vi "quadratic_eq_solve.vi"(2 "C":dbl, 3 "B":dbl, 4 "A":dbl) -> (0 "x2":dbl, 1 "x1":dbl)   [LabVIEW 2018]
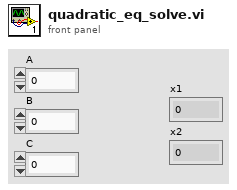
[diagram p1: front panel]
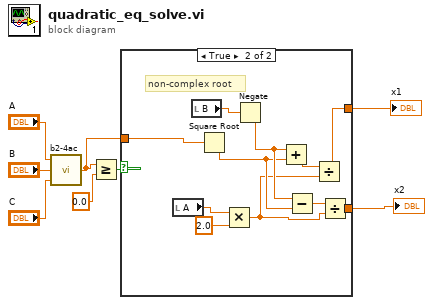
[diagram p0: block diagram]
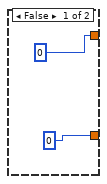
[diagram p2: hidden frame]
diagram:
  n1 = call "b2-4ac.vi"("C"="C", "B"="B", "A"="A") -> ("b2-4ac"=w2:dbl)
  n2 = Greater Or Equal?(x=w2, y=0.0) -> (x >= y?=w5:bool)
  n3 = case shown="True" w5 {
    tunnel: w2 -> [_ w21]
    tunnel: [0 w16] -> w4
    tunnel: [0 w11] -> w3
    frame False {
    }
    frame True {
      # "non-complex root"
      n4 = local read "A"() -> (w19:dbl)
      n5 = local read "B"() -> (w20:dbl)
      n6 = Square Root(x=w21) -> (sqrt(x)=w14:dbl)
      n7 = Multiply(x=w19, y=2.0) -> (x*y=w12:dbl)
      n8 = Negate(x=w20) -> (-x=w15:dbl)
      n9 = Add(x=w15, y=w14) -> (x+y=w17:dbl)
      n10 = Subtract(x=w15, y=w14) -> (x-y=w13:dbl)
      n11 = Divide(x=w17, y=w12) -> (x/y=w16:dbl)
      n12 = Divide(x=w13, y=w12) -> (x/y=w11:dbl)
    }
  }
  "x1" <- w4
  "x2" <- w3
